vi "transfer.vi"(0 "输入":string) -> (1 "待处理数据输出":u8[](array[numeric]), 2 "功能":u8, 3 "接收输出":bool)   [LabVIEW 2014]
panel:
  in  "枚举":enum16{"检测头0", "检测头1", "功能码", "长度和核对sum", "数据"}(ring)
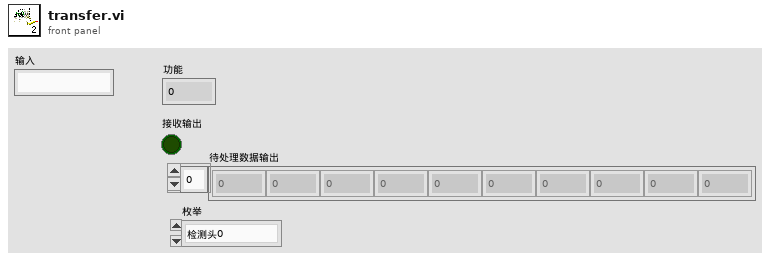
[diagram p1: front panel]
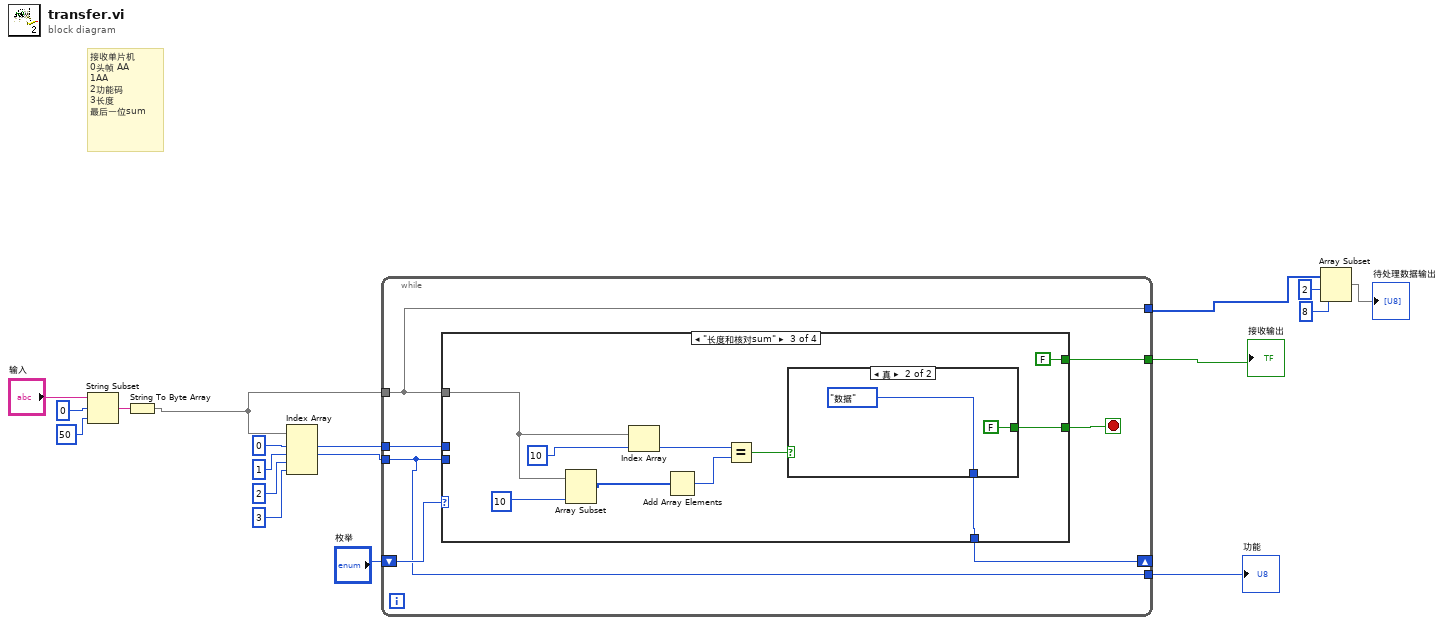
[diagram p0: block diagram]
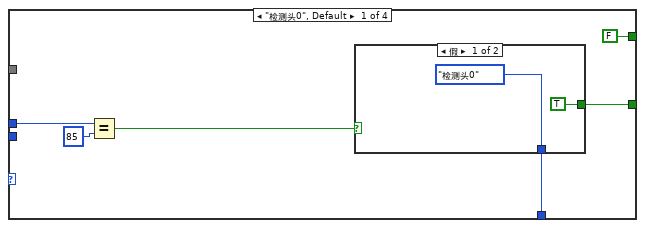
[diagram p2: hidden frame]
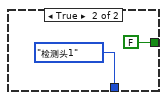
[diagram p3: hidden frame]
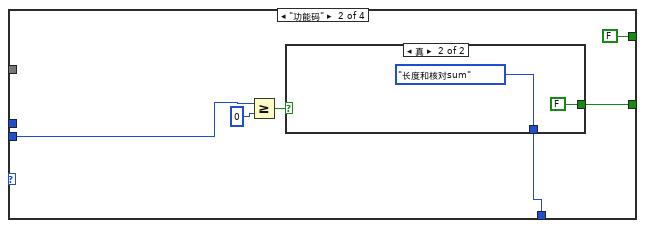
[diagram p4: hidden frame]
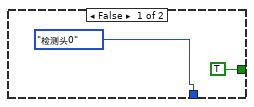
[diagram p5: hidden frame]
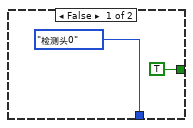
[diagram p6: hidden frame]
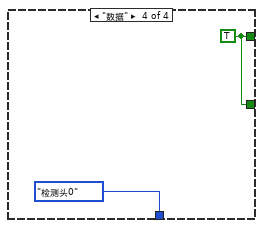
[diagram p7: hidden frame]
diagram:
  # "接收单片机\n0头帧 AA \n1AA\n2功能码\n3长度\n最后一位sum"
  n1 = String Subset(string="输入", offset (0)=0 ("长度（剩余）"), length (rest)=50 ("长度（剩余）")) -> (substring=w6:string)
  n2 = String To Byte Array(string=w6) -> (unsigned byte array=w5:u8[])
  n3 = Index Array(array=w5, index #1=0 ("长度（剩余）"), index #2=1 ("长度（剩余）"), index #3=2 ("索引"), index #4=3 ("索引")) -> (element #1=w14:u8, element #2=w12:u8)  [unwired: 2 out]
  n4 = while {
    tunnel: w14 -> [w24]
    shift-right: [w22] -> _
    shift-left: "枚举" -> [w23]
    tunnel: w12 -> [w19]
    tunnel: w5 -> [w20]
    tunnel: [w21] -> w11
    tunnel: [w20] -> w4
    tunnel: [w19] -> w10
    stop <- w25 stop-if-true
    n5 = case shown="\"长度和核对sum\"" w23 {
      tunnel: w24 -> [w29 _ _ _]
      tunnel: [FALSE ("布尔") FALSE ("布尔") FALSE ("布尔") w61] -> w21
      tunnel: [w27 w38 w52 w61] -> w25
      tunnel: [w26 w37 w48 enum16{"检测头0", "检测头1", "功能码", "长度和核对sum", "数据"}."检测头0" ("枚举")] -> w22
      tunnel: w19 -> [_ w36 _ _]
      tunnel: w20 -> [_ _ w49 _]
      frame "检测头0", Default {
        n6 = Equal?(x=w29, y=85 ("长度（剩余）")) -> (x = y?=w30:bool)
        n7 = case shown="假" w30 {
          tunnel: [TRUE FALSE ("布尔")] -> w27
          tunnel: [enum16{"检测头0", "检测头1", "功能码", "长度和核对sum", "数据"}."检测头0" ("枚举") enum16{"检测头0", "检测头1", "功能码", "长度和核对sum", "数据"}."检测头1" ("枚举")] -> w26
          frame False {
          }
          frame True {
          }
        }
      }
      frame "功能码" {
        n8 = Greater Or Equal?(x=w36, y=u8 0) -> (x >= y?=w40:bool)
        n9 = case shown="真" w40 {
          tunnel: [TRUE FALSE ("布尔")] -> w38
          tunnel: [enum16{"检测头0", "检测头1", "功能码", "长度和核对sum", "数据"}."检测头0" ("枚举") enum16{"检测头0", "检测头1", "功能码", "长度和核对sum", "数据"}."长度和核对sum" ("枚举")] -> w37
          frame False {
          }
          frame True {
          }
        }
      }
      frame "长度和核对sum" {
        n10 = Array Subset(array=w49, length=u8 10 ("y")) -> (w51:u8[])  [unwired: 1 in]
        n11 = Index Array(array=w49, index=u8 10 ("y")) -> (element=w50:u8)
        n12 = Add Array Elements(numeric array=w51) -> (sum=w55:u8)
        n13 = Equal?(x=w50, y=w55) -> (x = y?=w54:bool)
        n14 = case shown="真" w54 {
          tunnel: [TRUE FALSE ("布尔")] -> w52
          tunnel: [enum16{"检测头0", "检测头1", "功能码", "长度和核对sum", "数据"}."检测头0" ("枚举") enum16{"检测头0", "检测头1", "功能码", "长度和核对sum", "数据"}."数据" ("枚举")] -> w48
          frame False {
          }
          frame True {
          }
        }
      }
      frame "数据" {
        w61 = TRUE ("布尔")
      }
    }
  }
  "功能" <- w10
  "接收输出" <- w11
  n15 = Array Subset(array=w4, index=2 ("索引"), length=8 ("长度")) -> (→"待处理数据输出":u8[])
